vi "SMU calibration_Manual.vi"() -> ()   [LabVIEW 2020]
uses:
  <vilib>/Instr/_visa.llb/VISA Configure Serial Port (Instr).vi
  <vilib>/Analysis/NI_AALPro.lvlib
panel:
  out "output cal":dbl
  out "NewVal":bool
  out "tmp data":string
  out "Array":T1(array[cluster]) {"Output level" format="%.7f"; "Voltage" format="%.7f"; "Measurement" format="%.7f"}
  out "Array 3":bool[](array[boolean])
  out "Array 2":i32[](array[numeric])
  out "Unit":string
  in  "Output Value":dbl format="%.3f"
  in  "set Output":bool
  in  "Range":u16(ring) items=["1A", "100mA", "10mA", "1mA", "100uA", "10uA", "1uA"]
  in  "set range":bool
  in  "set mode":bool
  in  "Mode":bool
  out "test":bool
  out "extra buffer":string
  out "Write mode":bool
  in  "Enable":bool
  in  "Ring":u16(ring)=1 items=["Channel 1"=1, "Channel 2"=2, "Channel 3"=3, "Channel 4"=4]
  out "Range":string
  out "VI mode":string
  out "Enable":string
  out "Current":dbl
  out "Voltage":dbl
  out "Output level":dbl
  out "SMU Channel":string
  out "read buffer":string
  in  "VISA resource name":refnum<visa-resource-name>
  in  "stop":bool
  in  "set En":bool
  in  "String":string
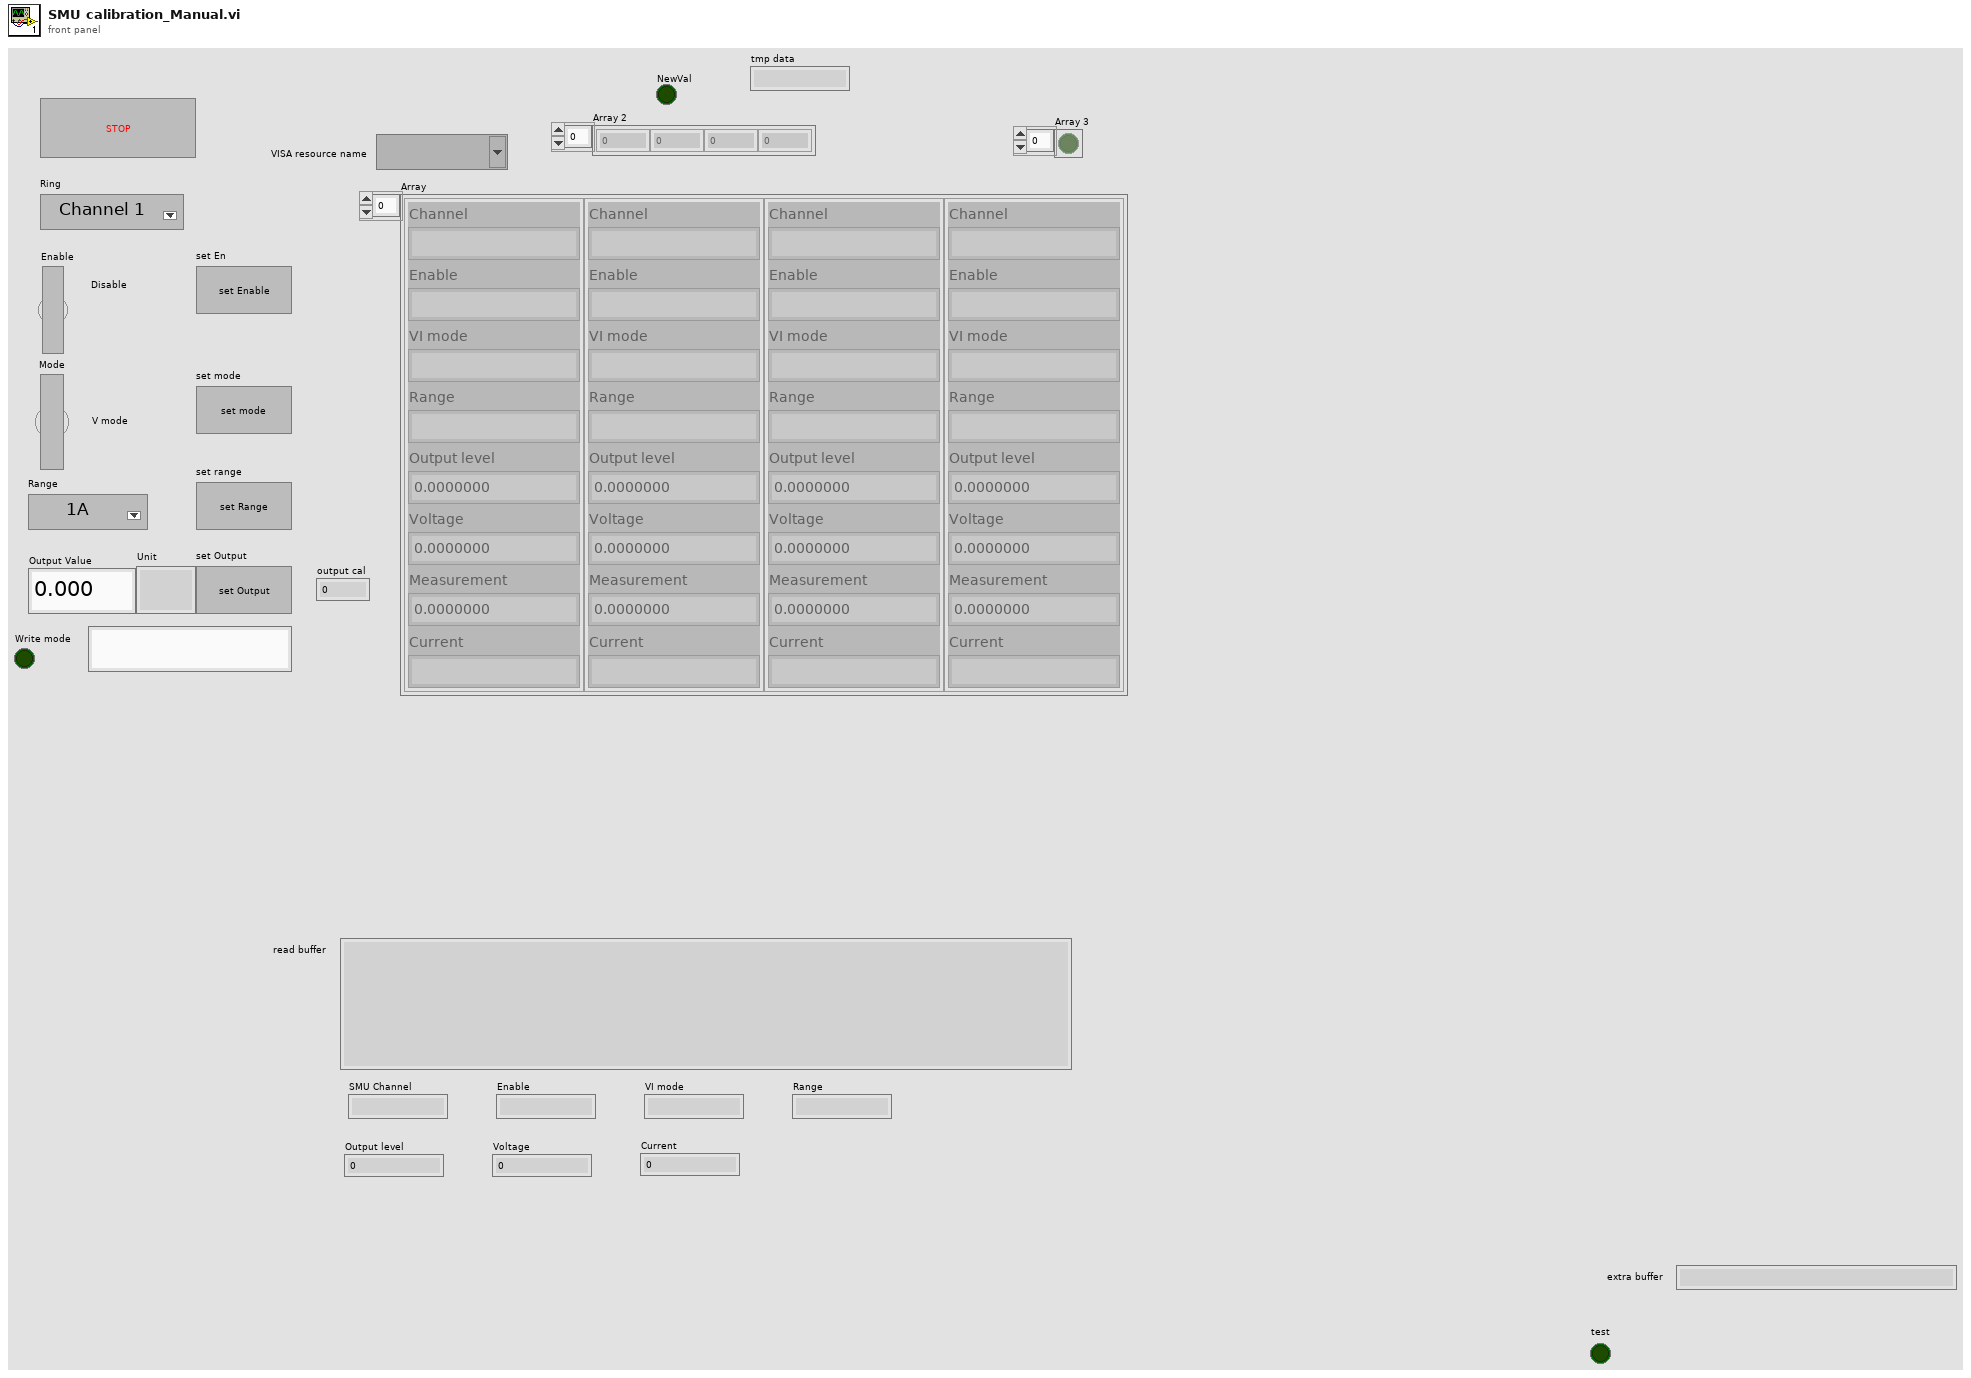
[diagram p1: front panel]
types:
  T1 = cluster{"Channel":string, "Enable":string, "VI mode":string, "Range":string, "Output level":dbl, "Voltage":dbl, "Measurement":dbl, "Current":string}[]
  T2 = cluster{"trimmed string":string, "Enable":string, "VI mode":string, "output string":string, dbl, dbl, dbl, string}
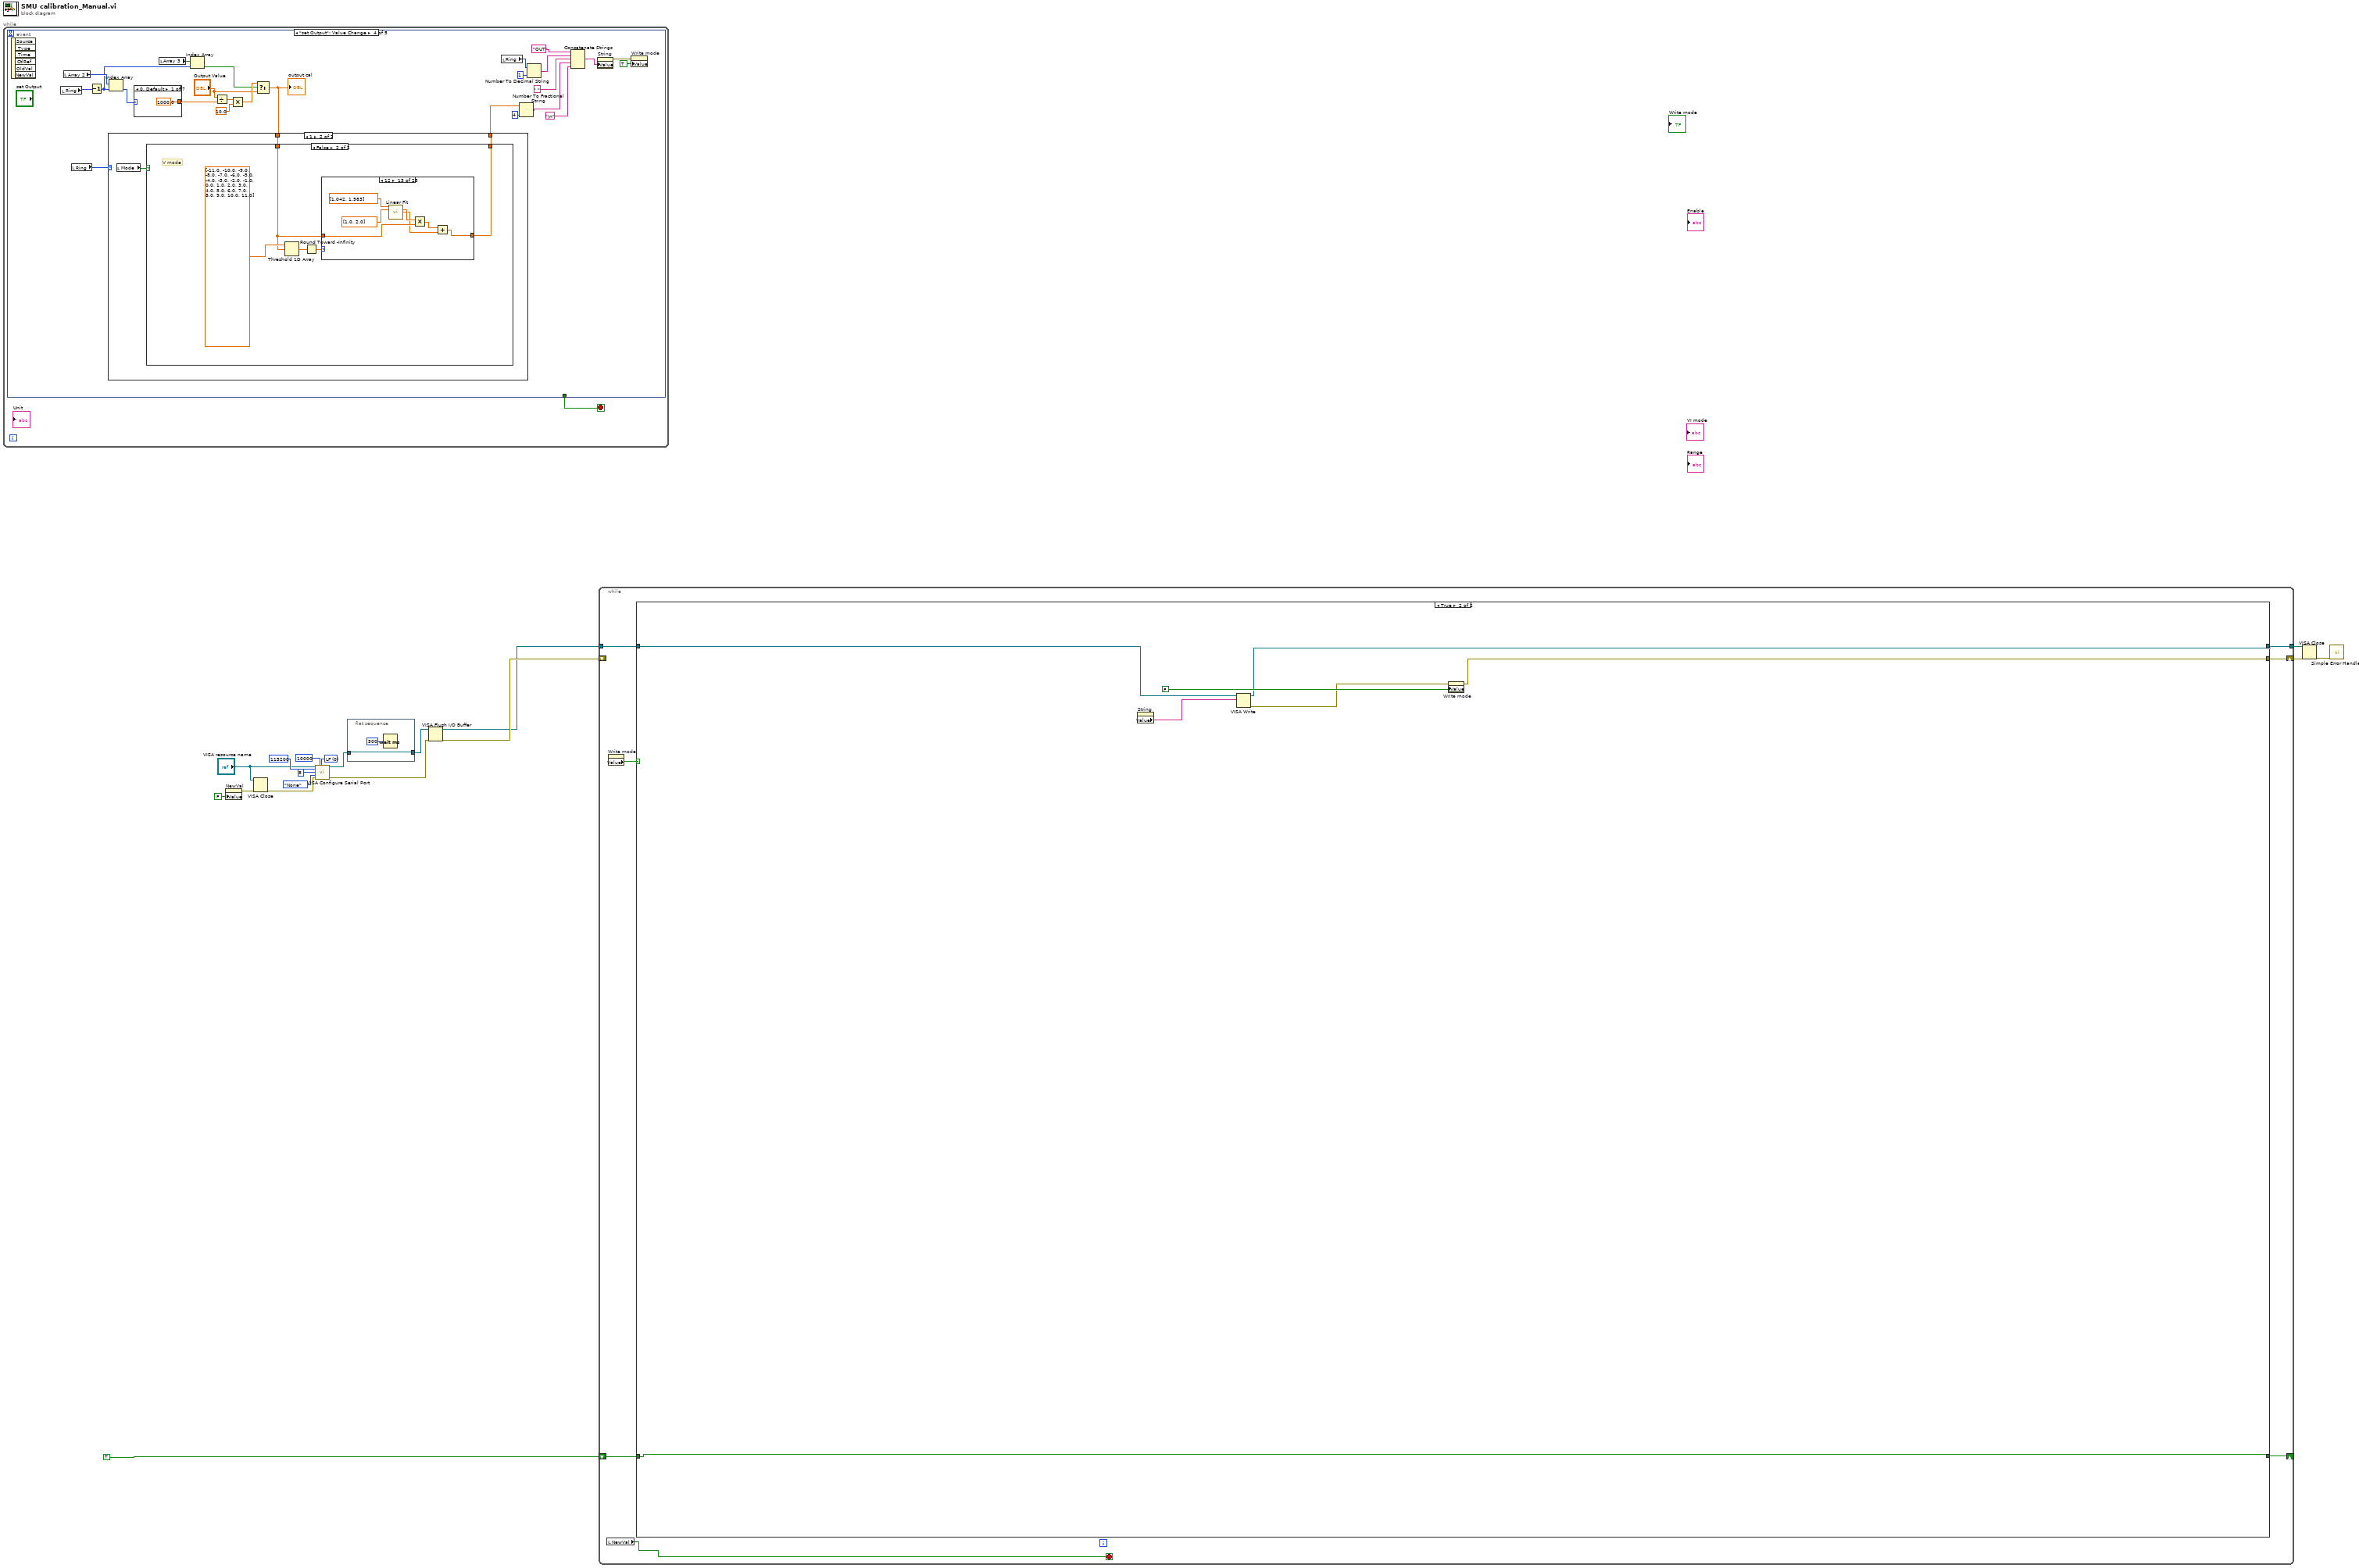
[diagram p0: block diagram]
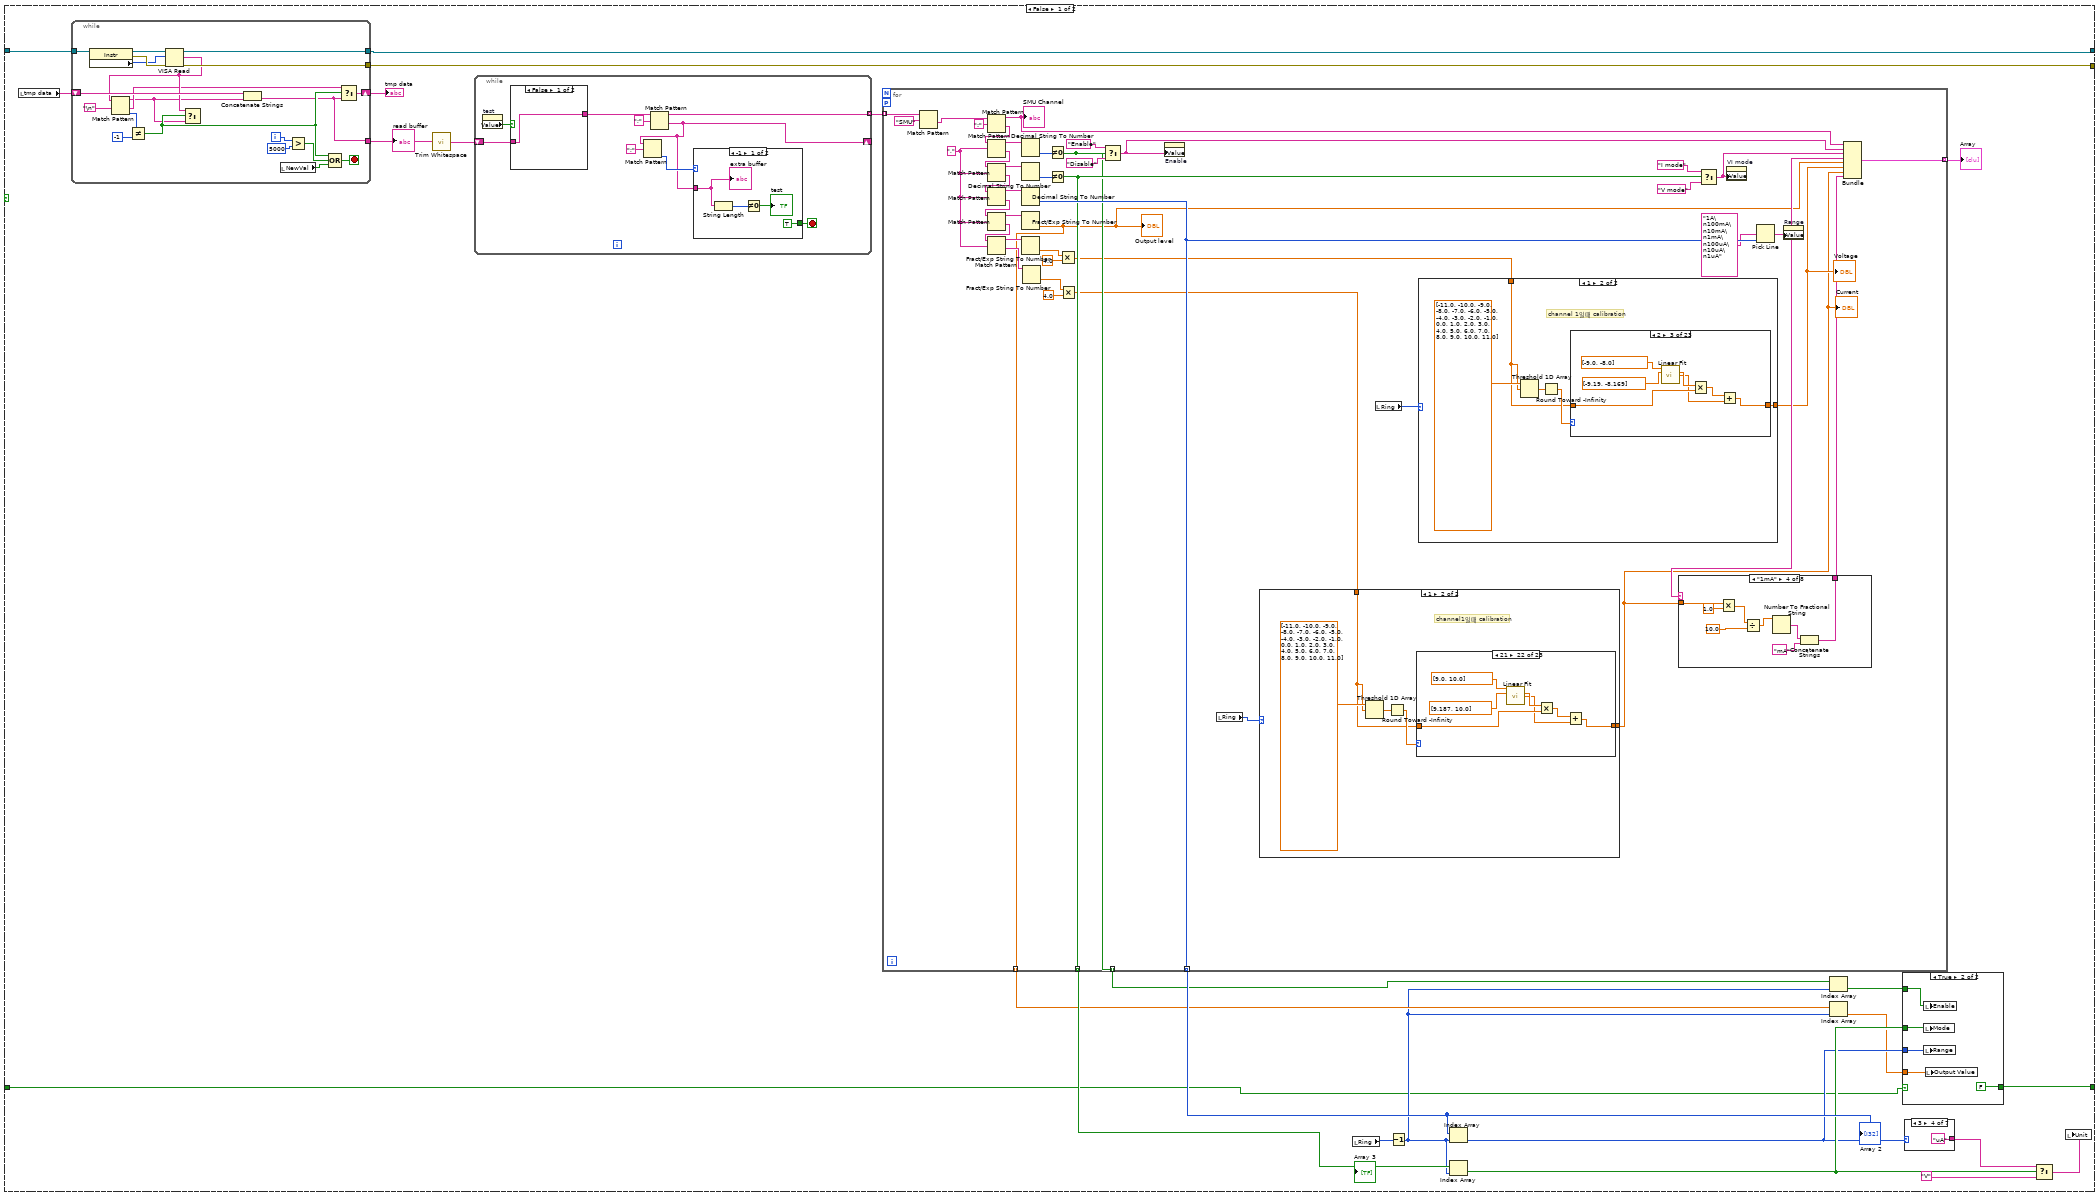
[diagram p2: hidden frame]
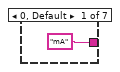
[diagram p4: hidden frame]
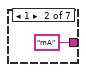
[diagram p5: hidden frame]
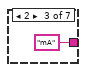
[diagram p6: hidden frame]
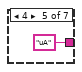
[diagram p7: hidden frame]
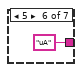
[diagram p8: hidden frame]
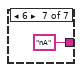
[diagram p9: hidden frame]
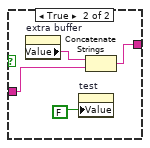
[diagram p10: hidden frame]
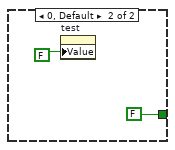
[diagram p11: hidden frame]
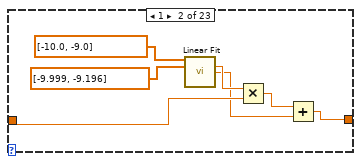
[diagram p14: hidden frame]
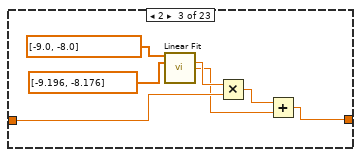
[diagram p15: hidden frame]
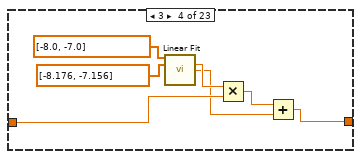
[diagram p16: hidden frame]
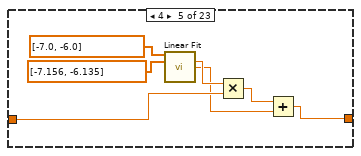
[diagram p17: hidden frame]
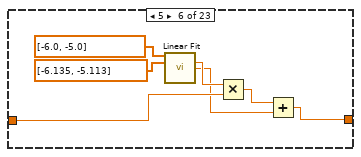
[diagram p18: hidden frame]
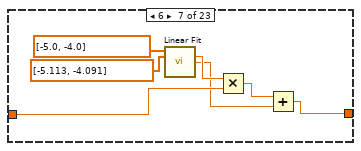
[diagram p19: hidden frame]
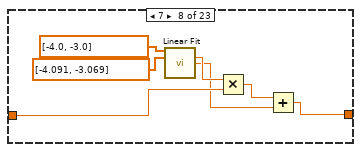
[diagram p20: hidden frame]
diagram:
  w16 = u16 0 items=["LF"]
  n1 = while {
    stop <- w19 stop-if-true
    n2 = event shown="[3] \"set Output\": Value Change" {
      selector: _ -> [_ _ _ _ _]
      dyn-events: _ -> [_ _ _ _ _]
      timeout: _ -> [_ _ _ _ _]
      tunnel: [_ _ _ _ w395] -> w19
      event "set En": Value Change {
        n3 = event-data() -> ()  [unwired: 1 in, 6 out]
        n4 = Boolean To (0,1)(Boolean="Enable") -> (0, 1=w31:i16)
        n5 = Number To Decimal String(number="Ring", width (-)=i16 1) -> (decimal integer string=w29:string)
        n6 = Number To Decimal String(number=w31, width (-)=i16 1) -> (decimal integer string=w32:string)
        n7 = Concatenate Strings("ENA", w29, " " ("string"), w32, "\n") -> (w20:string)
        n8 = property on="String" class="Str"("Value"=w20) -> (error out=w22:errorcluster)  [unwired: 2 in, 1 out]
        n9 = property on="Write mode" class="Bool (strict)"(error in=w22, "Value"=TRUE ("Write mode")) -> ()  [unwired: 1 in, 2 out]
      }
      event "set mode": Value Change {
        n10 = event-data() -> ()  [unwired: 1 in, 6 out]
        n11 = local read "Ring"() -> (w45:u16)
        n12 = Boolean To (0,1)(Boolean="Mode") -> (0, 1=w43:i16)
        n13 = Number To Decimal String(number=w45, width (-)=i16 1) -> (decimal integer string=w41:string)
        n14 = Number To Decimal String(number=w43, width (-)=i16 1) -> (decimal integer string=w44:string)
        n15 = Concatenate Strings("VIM", w41, " " ("string"), w44, "\n") -> (w39:string)
        n16 = property on="String" class="Str"("Value"=w39) -> (error out=w40:errorcluster)  [unwired: 2 in, 1 out]
        n17 = property on="Write mode" class="Bool (strict)"(error in=w40, "Value"=TRUE ("Write mode")) -> ()  [unwired: 1 in, 2 out]
      }
      event "set range": Value Change {
        n18 = event-data() -> ()  [unwired: 1 in, 6 out]
        n19 = local read "Ring"() -> (w56:u16)
        n20 = Number To Decimal String(number=w56, width (-)=i16 1) -> (decimal integer string=w54:string)
        n21 = Number To Decimal String(number="Range", width (-)=i16 1) -> (decimal integer string=w55:string)
        n22 = Concatenate Strings("RAN", w54, " " ("string"), w55, "\n") -> (w52:string)
        n23 = property on="String" class="Str"("Value"=w52) -> (error out=w53:errorcluster)  [unwired: 2 in, 1 out]
        n24 = property on="Write mode" class="Bool (strict)"(error in=w53, "Value"=TRUE ("Write mode")) -> ()  [unwired: 1 in, 2 out]
      }
      event "set Output": Value Change {
        n25 = event-data() -> ()  [unwired: 1 in, 6 out]
        n26 = local read "Ring"() -> (w68:u16)
        n27 = local read "Array 2"() -> (w67:i32[])
        n28 = local read "Ring"() -> (w58:u16)
        n29 = Decrement(x=w68) -> (x-1=w61:u16)
        n30 = Index Array(array=w67, index=w61) -> (element=w66:i32)
        n31 = case shown="0, Default" w66 {
          tunnel: [1000.0 100.0 10.0 1000.0 100.0 10.0 1.0] -> w69
          frame 0, Default {
          }
          frame 1 {
          }
          frame 2 {
          }
          frame 3 {
          }
          frame 4 {
          }
          frame 5 {
          }
          frame 6 {
          }
        }
        n32 = local read "Array 3"() -> (w63:bool[])
        n33 = Index Array(array=w63, index=w61) -> (element=w62:bool)
        n34 = Divide(x="Output Value", y=w69) -> (x/y=w70:dbl)
        n35 = Multiply(x=w70, y=10.0) -> (x*y=w65:dbl)
        n36 = Select(t=w65, s=w62, f="Output Value") -> (s? t:f=w60:dbl)
        "output cal" <- w60
        n37 = case shown="1" w58 {
          tunnel: w60 -> [w83 w86]
          tunnel: [w83 w85] -> w59
          frame 0, Default {
          }
          frame 1 {
            n38 = local read "Mode"() -> (w84:bool)
            n39 = case shown="False" w84 {
              tunnel: w86 -> [w88 w235]
              tunnel: [w87 w234] -> w85
              frame True {
                # "I mode"
                n40 = local read "Range"() -> (w89:u16)
                n41 = case shown="1" w89 {
                  tunnel: w88 -> [w90 w95 w119 w148 w177 w206]
                  tunnel: [w90 w94 w118 w147 w176 w205] -> w87
                  frame 0, Default {
                  }
                  frame 1 {
                    # "100mA일 경우"
                    n42 = Threshold 1D Array(2:w95, 3:dbl[] [-4.0, -3.5, -3.0, -2.0, -1.0, 0.0, 1.0, 2.0, 3.0, 4.0, 5.0, 6.0, 6.0]) -> (0:w92:dbl)  [unwired: 1 in]
                    n43 = Round Toward -Infinity(1:w92) -> (0:w91:dbl)
                    n44 = case shown="7" w91 {
                      tunnel: w95 -> [w96 w98 w100 w102 w104 w106 w108 w110 w112 w114 w116 w117]
                      tunnel: [w96 w97 w99 w101 w103 w105 w107 w109 w111 w113 w115 w117] -> w94
                      frame 0, Default {
                      }
                      frame 1 {
                        n45 = expression code="1.07 *x - 0.014"(w98) -> (w97:dbl)
                      }
                      frame 2 {
                        n46 = expression code="1.071* x - 0.011"(w100) -> (w99:dbl)
                      }
                      frame 3 {
                        n47 = expression code="1.071 *x - 0.011"(w102) -> (w101:dbl)
                      }
                      frame 4 {
                        n48 = expression code="1.075 * x - 0.007"(w104) -> (w103:dbl)
                      }
                      frame 5 {
                        n49 = expression code="1.069 *x - 0.007"(w106) -> (w105:dbl)
                      }
                      frame 6 {
                        n50 = expression code="1.071* x - 0.009"(w108) -> (w107:dbl)
                      }
                      frame 7 {
                        n51 = expression code="1.07* x - 0.007"(w110) -> (w109:dbl)
                      }
                      frame 8 {
                        n52 = expression code="1.069 *x - 0.004"(w112) -> (w111:dbl)
                      }
                      frame 9 {
                        n53 = expression code="1.07 *x - 0.008"(w114) -> (w113:dbl)
                      }
                      frame 10 {
                        n54 = expression code="1.07 *x - 0.008"(w116) -> (w115:dbl)
                      }
                      frame 11 {
                      }
                    }
                  }
                  frame 2 {
                    # "10mA일 경우"
                    n55 = Threshold 1D Array(2:w119, 3:dbl[] [-6.0, -5.0, -4.0, -3.0, -2.0, -1.0, 0.0, 1.0, 2.0, 3.0, 4.0, 5.0, 6.0]) -> (0:w122:dbl)  [unwired: 1 in]
                    n56 = Round Toward -Infinity(1:w122) -> (0:w121:dbl)
                    n57 = case shown="0, Default" w121 {
                      tunnel: w119 -> [w123 w125 w127 w129 w131 w133 w135 w137 w139 w141 w143 w145 w146]
                      tunnel: [w123 w124 w126 w128 w130 w132 w134 w136 w138 w140 w142 w144 w146] -> w118
                      frame 0, Default {
                      }
                      frame 1 {
                        n58 = expression code="1.043 * x - 0.01"(w125) -> (w124:dbl)
                      }
                      frame 2 {
                        n59 = expression code="1.043 * x - 0.01"(w127) -> (w126:dbl)
                      }
                      frame 3 {
                        n60 = expression code="1.042 * x - 0.013"(w129) -> (w128:dbl)
                      }
                      frame 4 {
                        n61 = expression code="1.043 * x - 0.011"(w131) -> (w130:dbl)
                      }
                      frame 5 {
                        n62 = expression code="1.044 * x - 0.01"(w133) -> (w132:dbl)
                      }
                      frame 6 {
                        n63 = expression code="1.045 * x - 0.01"(w135) -> (w134:dbl)
                      }
                      frame 7 {
                        n64 = expression code="1.042 * x - 0.007"(w137) -> (w136:dbl)
                      }
                      frame 8 {
                        n65 = expression code="1.043 * x - 0.009"(w139) -> (w138:dbl)
                      }
                      frame 9 {
                        n66 = expression code="1.042 * x - 0.006"(w141) -> (w140:dbl)
                      }
                      frame 10 {
                        n67 = expression code="1.041 * x - 0.002"(w143) -> (w142:dbl)
                      }
                      frame 11 {
                        n68 = expression code="1.043 * x - 0.012"(w145) -> (w144:dbl)
                      }
                      frame 12 {
                      }
                    }
                  }
                  frame 3 {
                    # "1mA 경우"
                    n69 = Threshold 1D Array(2:w148, 3:dbl[] [-6.0, -5.0, -4.0, -3.0, -2.0, -1.0, 0.0, 1.0, 2.0, 3.0, 4.0, 5.0, 6.0]) -> (0:w151:dbl)  [unwired: 1 in]
                    n70 = Round Toward -Infinity(1:w151) -> (0:w150:dbl)
                    n71 = case shown="12" w150 {
                      tunnel: w148 -> [w152 w154 w156 w158 w160 w162 w164 w166 w168 w170 w172 w174 w175]
                      tunnel: [w152 w153 w155 w157 w159 w161 w163 w165 w167 w169 w171 w173 w175] -> w147
                      frame 0, Default {
                      }
                      frame 1 {
                        n72 = expression code="1.043 *x - 0.009"(w154) -> (w153:dbl)
                      }
                      frame 2 {
                        n73 = expression code="1.042 *x - 0.013"(w156) -> (w155:dbl)
                      }
                      frame 3 {
                        n74 = expression code="1.042 *x - 0.013"(w158) -> (w157:dbl)
                      }
                      frame 4 {
                        n75 = expression code="1.043* x - 0.011"(w160) -> (w159:dbl)
                      }
                      frame 5 {
                        n76 = expression code="1.042* x - 0.012"(w162) -> (w161:dbl)
                      }
                      frame 6 {
                        n77 = expression code="1.046 *x - 0.012"(w164) -> (w163:dbl)
                      }
                      frame 7 {
                        n78 = expression code="1.042 *x - 0.008"(w166) -> (w165:dbl)
                      }
                      frame 8 {
                        n79 = expression code="1.042 *x - 0.008"(w168) -> (w167:dbl)
                      }
                      frame 9 {
                        n80 = expression code="1.043 *x - 0.011"(w170) -> (w169:dbl)
                      }
                      frame 10 {
                        n81 = expression code="1.041 *x - 0.003"(w172) -> (w171:dbl)
                      }
                      frame 11 {
                        n82 = expression code="1.042 *x - 0.008"(w174) -> (w173:dbl)
                      }
                      frame 12 {
                      }
                    }
                  }
                  frame 4 {
                    # "100uA 경우"
                    n83 = Threshold 1D Array(2:w177, 3:dbl[] [-6.0, -5.0, -4.0, -3.0, -2.0, -1.0, 0.0, 1.0, 2.0, 3.0, 4.0, 5.0, 6.0]) -> (0:w180:dbl)  [unwired: 1 in]
                    n84 = Round Toward -Infinity(1:w180) -> (0:w179:dbl)
                    n85 = case shown="12" w179 {
                      tunnel: w177 -> [w181 w183 w185 w187 w189 w191 w193 w195 w197 w199 w201 w203 w204]
                      tunnel: [w181 w182 w184 w186 w188 w190 w192 w194 w196 w198 w200 w202 w204] -> w176
                      frame 0, Default {
                      }
                      frame 1 {
                        n86 = expression code="1.046 *x - 0.001"(w183) -> (w182:dbl)
                      }
                      frame 2 {
                        n87 = expression code="1.042* x - 0.017"(w185) -> (w184:dbl)
                      }
                      frame 3 {
                        n88 = expression code="1.044 *x - 0.011"(w187) -> (w186:dbl)
                      }
                      frame 4 {
                        n89 = expression code="1.042 *x - 0.015"(w189) -> (w188:dbl)
                      }
                      frame 5 {
                        n90 = expression code="1.043* x - 0.014"(w191) -> (w190:dbl)
                      }
                      frame 6 {
                        n91 = expression code="1.043* x - 0.014"(w193) -> (w192:dbl)
                      }
                      frame 7 {
                        n92 = expression code="1.042 *x - 0.013"(w195) -> (w194:dbl)
                      }
                      frame 8 {
                        n93 = expression code="1.041* x - 0.011"(w197) -> (w196:dbl)
                      }
                      frame 9 {
                        n94 = expression code="1.041* x - 0.011"(w199) -> (w198:dbl)
                      }
                      frame 10 {
                        n95 = expression code="1.041* x - 0.011"(w201) -> (w200:dbl)
                      }
                      frame 11 {
                        n96 = expression code="1.042 *x - 0.008"(w203) -> (w202:dbl)
                      }
                      frame 12 {
                      }
                    }
                  }
                  frame 5 {
                    # "10uA 경우"
                    n97 = Threshold 1D Array(2:w206, 3:dbl[] [-6.0, -5.0, -4.0, -3.0, -2.0, -1.0, 0.0, 1.0, 2.0, 3.0, 4.0, 5.0, 6.0]) -> (0:w209:dbl)  [unwired: 1 in]
                    n98 = Round Toward -Infinity(1:w209) -> (0:w208:dbl)
                    n99 = case shown="12" w208 {
                      tunnel: w206 -> [w210 w212 w214 w216 w218 w220 w222 w224 w226 w228 w230 w232 w233]
                      tunnel: [w210 w211 w213 w215 w217 w219 w221 w223 w225 w227 w229 w231 w233] -> w205
                      frame 0, Default {
                      }
                      frame 1 {
                        n100 = expression code="1.045* x - 0.05"(w212) -> (w211:dbl)
                      }
                      frame 2 {
                        n101 = expression code="1.045 *x - 0.05"(w214) -> (w213:dbl)
                      }
                      frame 3 {
                        n102 = expression code="1.055 *x - 0.02"(w216) -> (w215:dbl)
                      }
                      frame 4 {
                        n103 = expression code="1.041 *x - 0.048"(w218) -> (w217:dbl)
                      }
                      frame 5 {
                        n104 = expression code="1.039 *x - 0.05"(w220) -> (w219:dbl)
                      }
                      frame 6 {
                        n105 = expression code="1.048 *x - 0.05"(w222) -> (w221:dbl)
                      }
                      frame 7 {
                        n106 = expression code="1.039* x - 0.041"(w224) -> (w223:dbl)
                      }
                      frame 8 {
                        n107 = expression code="1.045* x - 0.053"(w226) -> (w225:dbl)
                      }
                      frame 9 {
                        n108 = expression code="1.039 *x - 0.035"(w228) -> (w227:dbl)
                      }
                      frame 10 {
                        n109 = expression code="1.034 *x - 0.015"(w230) -> (w229:dbl)
                      }
                      frame 11 {
                        n110 = expression code="1.054* x - 0.115"(w232) -> (w231:dbl)
                      }
                      frame 12 {
                      }
                    }
                  }
                }
              }
              frame False {
                # "V mode"
                n111 = Threshold 1D Array(2:w235, 3:dbl[] [-11.0, -10.0, -9.0, -8.0, -7.0, -6.0, -5.0, -4.0, -3.0, -2.0, -1.0, 0.0, 1.0, 2.0, 3.0, 4.0, 5.0, 6.0, 7.0, 8.0, 9.0, 10.0, 11.0]) -> (0:w238:dbl)  [unwired: 1 in]
                n112 = Round Toward -Infinity(1:w238) -> (0:w236:dbl)
                n113 = case shown="12" w236 {
                  tunnel: w235 -> [w239 w245 w252 w259 w266 w273 w280 w287 w294 w301 w306 w313 w320 w327 w334 w341 w348 w355 w362 w369 w376 w383 w387]
                  tunnel: [w239 w242 w249 w256 w263 w270 w277 w284 w291 w298 w303 w310 w317 w324 w331 w338 w345 w352 w359 w366 w373 w380 w387] -> w234
                  frame 0, Default {
                  }
                  frame 1 {
                    n114 = call <vilib>:"Linear Fit.vi"("Y"=dbl[] [-9.308, -8.367], "X"=dbl[] [-10.0, -9.0]) -> ("slope"=w246:dbl, "intercept"=w244:dbl)  [unwired: 9 in, 3 out]
                    n115 = Multiply(x=w246, y=w245) -> (x*y=w243:dbl)
                    n116 = Add(x=w243, y=w244) -> (x+y=w242:dbl)
                  }
                  frame 2 {
                    n117 = call <vilib>:"Linear Fit.vi"("Y"=dbl[] [-8.367, -7.427], "X"=dbl[] [-9.0, -8.0]) -> ("slope"=w253:dbl, "intercept"=w251:dbl)  [unwired: 9 in, 3 out]
                    n118 = Multiply(x=w253, y=w252) -> (x*y=w250:dbl)
                    n119 = Add(x=w250, y=w251) -> (x+y=w249:dbl)
                  }
                  frame 3 {
                    n120 = call <vilib>:"Linear Fit.vi"("Y"=dbl[] [-7.427, -6.486], "X"=dbl[] [-8.0, -7.0]) -> ("slope"=w260:dbl, "intercept"=w258:dbl)  [unwired: 9 in, 3 out]
                    n121 = Multiply(x=w260, y=w259) -> (x*y=w257:dbl)
                    n122 = Add(x=w257, y=w258) -> (x+y=w256:dbl)
                  }
                  frame 4 {
                    n123 = call <vilib>:"Linear Fit.vi"("Y"=dbl[] [-6.486, -5.545], "X"=dbl[] [-7.0, -6.0]) -> ("slope"=w267:dbl, "intercept"=w265:dbl)  [unwired: 9 in, 3 out]
                    n124 = Multiply(x=w267, y=w266) -> (x*y=w264:dbl)
                    n125 = Add(x=w264, y=w265) -> (x+y=w263:dbl)
                  }
                  frame 5 {
                    n126 = call <vilib>:"Linear Fit.vi"("Y"=dbl[] [-5.545, -4.604], "X"=dbl[] [-6.0, -5.0]) -> ("slope"=w274:dbl, "intercept"=w272:dbl)  [unwired: 9 in, 3 out]
                    n127 = Multiply(x=w274, y=w273) -> (x*y=w271:dbl)
                    n128 = Add(x=w271, y=w272) -> (x+y=w270:dbl)
                  }
                  frame 6 {
                    n129 = call <vilib>:"Linear Fit.vi"("Y"=dbl[] [-4.604, -3.664], "X"=dbl[] [-5.0, -4.0]) -> ("slope"=w281:dbl, "intercept"=w279:dbl)  [unwired: 9 in, 3 out]
                    n130 = Multiply(x=w281, y=w280) -> (x*y=w278:dbl)
                    n131 = Add(x=w278, y=w279) -> (x+y=w277:dbl)
                  }
                  frame 7 {
                    n132 = call <vilib>:"Linear Fit.vi"("Y"=dbl[] [-3.664, -2.723], "X"=dbl[] [-4.0, -3.0]) -> ("slope"=w288:dbl, "intercept"=w286:dbl)  [unwired: 9 in, 3 out]
                    n133 = Multiply(x=w288, y=w287) -> (x*y=w285:dbl)
                    n134 = Add(x=w285, y=w286) -> (x+y=w284:dbl)
                  }
                  frame 8 {
                    n135 = call <vilib>:"Linear Fit.vi"("Y"=dbl[] [-2.723, -1.782], "X"=dbl[] [-3.0, -2.0]) -> ("slope"=w295:dbl, "intercept"=w293:dbl)  [unwired: 9 in, 3 out]
                    n136 = Multiply(x=w295, y=w294) -> (x*y=w292:dbl)
                    n137 = Add(x=w292, y=w293) -> (x+y=w291:dbl)
                  }
                  frame 9 {
                    n138 = call <vilib>:"Linear Fit.vi"("Y"=dbl[] [-1.782, -0.841], "X"=dbl[] [-2.0, -1.0]) -> ("slope"=w302:dbl, "intercept"=w300:dbl)  [unwired: 9 in, 3 out]
                    n139 = Multiply(x=w302, y=w301) -> (x*y=w299:dbl)
                    n140 = Add(x=w299, y=w300) -> (x+y=w298:dbl)
                  }
                  frame 10 {
                    n141 = call <vilib>:"Linear Fit.vi"("Y"=dbl[] [-0.841, 0.1], "X"=dbl[] [-1.0, 0.0]) -> ("slope"=w307:dbl, "intercept"=w305:dbl)  [unwired: 9 in, 3 out]
                    n142 = Multiply(x=w307, y=w306) -> (x*y=w304:dbl)
                    n143 = Add(x=w304, y=w305) -> (x+y=w303:dbl)
                  }
                  frame 11 {
                    n144 = call <vilib>:"Linear Fit.vi"("Y"=dbl[] [0.1, 1.042], "X"=dbl[] [0.0, 1.0]) -> ("slope"=w314:dbl, "intercept"=w312:dbl)  [unwired: 9 in, 3 out]
                    n145 = Multiply(x=w314, y=w313) -> (x*y=w311:dbl)
                    n146 = Add(x=w311, y=w312) -> (x+y=w310:dbl)
                  }
                  frame 12 {
                    n147 = call <vilib>:"Linear Fit.vi"("Y"=dbl[] [1.042, 1.983], "X"=dbl[] [1.0, 2.0]) -> ("slope"=w321:dbl, "intercept"=w319:dbl)  [unwired: 9 in, 3 out]
                    n148 = Multiply(x=w321, y=w320) -> (x*y=w318:dbl)
                    n149 = Add(x=w318, y=w319) -> (x+y=w317:dbl)
                  }
                  frame 13 {
                    n150 = call <vilib>:"Linear Fit.vi"("Y"=dbl[] [1.983, 2.924], "X"=dbl[] [2.0, 3.0]) -> ("slope"=w328:dbl, "intercept"=w326:dbl)  [unwired: 9 in, 3 out]
                    n151 = Multiply(x=w328, y=w327) -> (x*y=w325:dbl)
                    n152 = Add(x=w325, y=w326) -> (x+y=w324:dbl)
                  }
                  frame 14 {
                    n153 = call <vilib>:"Linear Fit.vi"("Y"=dbl[] [2.924, 3.864], "X"=dbl[] [3.0, 4.0]) -> ("slope"=w335:dbl, "intercept"=w333:dbl)  [unwired: 9 in, 3 out]
                    n154 = Multiply(x=w335, y=w334) -> (x*y=w332:dbl)
                    n155 = Add(x=w332, y=w333) -> (x+y=w331:dbl)
                  }
                  frame 15 {
                    n156 = call <vilib>:"Linear Fit.vi"("Y"=dbl[] [3.864, 4.804], "X"=dbl[] [4.0, 5.0]) -> ("slope"=w342:dbl, "intercept"=w340:dbl)  [unwired: 9 in, 3 out]
                    n157 = Multiply(x=w342, y=w341) -> (x*y=w339:dbl)
                    n158 = Add(x=w339, y=w340) -> (x+y=w338:dbl)
                  }
                  frame 16 {
                    n159 = call <vilib>:"Linear Fit.vi"("Y"=dbl[] [4.804, 5.745], "X"=dbl[] [5.0, 6.0]) -> ("slope"=w349:dbl, "intercept"=w347:dbl)  [unwired: 9 in, 3 out]
                    n160 = Multiply(x=w349, y=w348) -> (x*y=w346:dbl)
                    n161 = Add(x=w346, y=w347) -> (x+y=w345:dbl)
                  }
                  frame 17 {
                    n162 = call <vilib>:"Linear Fit.vi"("Y"=dbl[] [5.745, 6.686], "X"=dbl[] [6.0, 7.0]) -> ("slope"=w356:dbl, "intercept"=w354:dbl)  [unwired: 9 in, 3 out]
                    n163 = Multiply(x=w356, y=w355) -> (x*y=w353:dbl)
                    n164 = Add(x=w353, y=w354) -> (x+y=w352:dbl)
                  }
                  frame 18 {
                    n165 = call <vilib>:"Linear Fit.vi"("Y"=dbl[] [6.686, 7.627], "X"=dbl[] [7.0, 8.0]) -> ("slope"=w363:dbl, "intercept"=w361:dbl)  [unwired: 9 in, 3 out]
                    n166 = Multiply(x=w363, y=w362) -> (x*y=w360:dbl)
                    n167 = Add(x=w360, y=w361) -> (x+y=w359:dbl)
                  }
                  frame 19 {
                    n168 = call <vilib>:"Linear Fit.vi"("Y"=dbl[] [7.627, 8.567], "X"=dbl[] [8.0, 9.0]) -> ("slope"=w370:dbl, "intercept"=w368:dbl)  [unwired: 9 in, 3 out]
                    n169 = Multiply(x=w370, y=w369) -> (x*y=w367:dbl)
                    n170 = Add(x=w367, y=w368) -> (x+y=w366:dbl)
                  }
                  frame 20 {
                    n171 = call <vilib>:"Linear Fit.vi"("Y"=dbl[] [8.567, 9.507], "X"=dbl[] [9.0, 10.0]) -> ("slope"=w377:dbl, "intercept"=w375:dbl)  [unwired: 9 in, 3 out]
                    n172 = Multiply(x=w377, y=w376) -> (x*y=w374:dbl)
                    n173 = Add(x=w374, y=w375) -> (x+y=w373:dbl)
                  }
                  frame 21 {
                    n174 = call <vilib>:"Linear Fit.vi"("Y"=dbl[] [8.567, 9.507], "X"=dbl[] [9.0, 10.0]) -> ("slope"=w384:dbl, "intercept"=w382:dbl)  [unwired: 9 in, 3 out]
                    n175 = Multiply(x=w384, y=w383) -> (x*y=w381:dbl)
                    n176 = Add(x=w381, y=w382) -> (x+y=w380:dbl)
                  }
                  frame 22 {
                  }
                }
              }
            }
          }
        }
        n177 = local read "Ring"() -> (w81:u16)
        n178 = Number To Fractional String(number=w59, precision (6)=i16 4) -> (F-format string=w82:string)  [unwired: 2 in]
        n179 = Number To Decimal String(number=w81, width (-)=i16 1) -> (decimal integer string=w80:string)
        n180 = Concatenate Strings("OUT", w80, " " ("string"), w82, "\n") -> (w78:string)
        n181 = property on="String" class="Str"("Value"=w78) -> (error out=w79:errorcluster)  [unwired: 2 in, 1 out]
        n182 = property on="Write mode" class="Bool (strict)"(error in=w79, "Value"=TRUE ("Write mode")) -> ()  [unwired: 1 in, 2 out]
      }
      event "stop": Value Change {
        n183 = event-data() -> ("NewVal"=w395:bool)  [unwired: 1 in, 5 out]
        "NewVal" <- w395
      }
    }
  }
  n184 = property on="NewVal" class="Bool (strict)"("Value"=FALSE ("NewVal")) -> (error out=w2:errorcluster)  [unwired: 2 in, 1 out]
  n185 = VISA Close(VISA resource name="VISA resource name", error in (no error)=w2) -> (error out=w4:errorcluster)
  n186 = call-poly "VISA Configure Serial Port"("VISA resource name"="VISA resource name", "timeout (10sec)"=u32 10000, "termination char\n(0xA = '\\n' = LF)"=w16, "baud rate (9600)"=u32 115200, "data bits (8)"=u16 8, "parity (0:none)"=enum16{"None", "Odd", "Even", "Mark", "Space"}."None", "error in (no error)"=w4) -> ("VISA resource name out"=w10:refnum<visa-resource-name>, "error out"=w8:errorcluster)  [unwired: 7 in]
  n187 = flat-sequence {
    tunnel: [w396] -> w9
    tunnel: w10 -> [w396]
    frame #0 {
      n188 = Wait (ms)(milliseconds to wait=u32 500 ("대기 시간(ms)")) -> ()  [unwired: 1 out]
    }
  }
  n189 = VISA Flush I/O Buffer(VISA resource name=w9, error in (no error)=w8) -> (VISA resource name out=w6:refnum<visa-resource-name>, error out=w7:errorcluster)  [unwired: 1 in]
  n190 = while {
    tunnel: [w403] -> w18
    shift-right: [w404] -> w12
    shift-left: w7 -> [_]
    tunnel: w6 -> [w402]
    shift-right: [w399] -> _
    shift-left: TRUE -> [w400]
    stop <- w398 stop-if-true
    n191 = local read "NewVal"() -> (w398:bool)
    n192 = property on="Write mode" class="Bool (strict)"() -> ("Value"=w401:bool)  [unwired: 2 in, 2 out]
    n193 = case shown="True" w401 {
      tunnel: [w420 w894] -> w404
      tunnel: [w419 w895] -> w403
      tunnel: w402 -> [w421 w898]
      tunnel: w400 -> [w409 w893]
      tunnel: [w408 w893] -> w399
      frame False {
        n194 = local read "tmp data"() -> (w418:string)
        n195 = while {
          tunnel: w421 -> [w447]
          tunnel: [w455] -> w420
          tunnel: [w454] -> w419
          shift-right: [w453] -> w417
          shift-left: w418 -> [w452]
          tunnel: [w437] -> w406
          i -> [w450]
          stop <- w451 stop-if-true
          n196 = property class="Instr"(reference=w447) -> (reference out=w446:refnum<visa-resource-name>, error out=w445:errorcluster, "Serial Settings:Number of Bytes at Serial Port"=w444:u32)  [unwired: 1 in]
          n197 = VISA Read(VISA resource name=w446, byte count=w444, error in (no error)=w445) -> (VISA resource name out=w454:refnum<visa-resource-name>, read buffer=w439:string, error out=w455:errorcluster)  [unwired: 1 out]
          n198 = Match Pattern(string=w439, regular expression="\n") -> (before substring=w435:string, after substring=w438:string, offset past match=w442:i32)  [unwired: 1 in, 1 out]
          n199 = Not Equal?(x=w442, y=-1) -> (x != y?=w440:bool)
          n200 = Select(t=w439, s=w440, f=w435) -> ()  [unwired: 1 out]
          n201 = Concatenate Strings(w452, w435) -> (w437:string)
          n202 = local read "NewVal"() -> (w436:bool)
          n203 = Greater?(x=w450, y=5000) -> (0:w448:bool)
          n204 = Compound Arithmetic op=OR(w440, w448, w436) -> (w451:bool)
          n205 = Select(t=w438, s=w440, f=w437) -> (s? t:f=w453:string)
        }
        "read buffer" <- w406
        "tmp data" <- w417
        n206 = call <vilib>:"Trim Whitespace.vi"("string"=w406) -> ("trimmed string"=w407:string)  [unwired: 1 in]
        n207 = while {
          shift-right: [w463] -> _
          shift-left: w407 -> [w466]
          tunnel: [w470] -> w428 mode=indexing
          stop <- w464 stop-if-true
          n208 = property on="test" class="Bool (strict)"() -> ("Value"=w467:bool)  [unwired: 2 in, 2 out]
          n209 = case shown="False" w467 {
            tunnel: w466 -> [w472 w475]
            tunnel: [w472 w474] -> w465
            frame False {
            }
            frame True {
              n210 = property on="extra buffer" class="Str"() -> ("Value"=w476:string)  [unwired: 2 in, 2 out]
              n211 = property on="test" class="Bool (strict)"("Value"=FALSE) -> ()  [unwired: 2 in, 2 out]
              n212 = Concatenate Strings(w476, w475) -> (w474:string)
            }
          }
          n213 = Match Pattern(string=w465, regular expression=";" ("search string")) -> (before substring=w470:string, after substring=w463:string)  [unwired: 1 in, 2 out]
          n214 = Match Pattern(string=w463, regular expression=";" ("search string")) -> (offset past match=w468:i32)  [unwired: 1 in, 3 out]
          n215 = case shown="-1" w468 {
            tunnel: w463 -> [w479 _]
            tunnel: [TRUE FALSE] -> w464
            frame -1 {
              n216 = String Length(string=w479) -> (length=w478:i32)
              n217 = Not Equal To 0?(x=w478) -> (x != 0?=→"test":bool)
              "extra buffer" <- w479
            }
            frame 0, Default {
              n218 = property on="test" class="Bool (strict)"("Value"=FALSE) -> ()  [unwired: 2 in, 2 out]
            }
          }
        }
        n219 = for {
          tunnel: [w525] -> w405 mode=indexing
          tunnel: w428 -> [w500] mode=indexing
          workers-P: _ -> [_]
          tunnel: [w495] -> w426 mode=indexing
          tunnel: [w494] -> w425 mode=indexing
          tunnel: [w490] -> w416 mode=indexing
          tunnel: [w489] -> w412 mode=indexing
          w516 = "," ("search string")
          n220 = Match Pattern(string=w500, regular expression="SMU") -> (after substring=w522:string)  [unwired: 1 in, 3 out]
          n221 = Match Pattern(string=w522, regular expression=":" ("search string")) -> (before substring=w501:string, after substring=w521:string)  [unwired: 1 in, 2 out]
          "SMU Channel" <- w501
          n222 = Match Pattern(string=w521, regular expression=w516) -> (before substring=w515:string, after substring=w520:string)  [unwired: 1 in, 2 out]
          n223 = Match Pattern(string=w520, regular expression=w516) -> (before substring=w510:string, after substring=w518:string)  [unwired: 1 in, 2 out]
          n224 = Match Pattern(string=w518, regular expression=w516) -> (before substring=w511:string, after substring=w519:string)  [unwired: 1 in, 2 out]
          n225 = Match Pattern(string=w519, regular expression=w516) -> (before substring=w512:string, after substring=w517:string)  [unwired: 1 in, 2 out]
          n226 = Match Pattern(string=w517, regular expression=w516) -> (before substring=w513:string, after substring=w514:string)  [unwired: 1 in, 2 out]
          n227 = Decimal String To Number(string=w515) -> (number=w509:i32)  [unwired: 2 in, 1 out]
          n228 = Decimal String To Number(string=w510) -> (number=w508:i32)  [unwired: 2 in, 1 out]
          n229 = Decimal String To Number(string=w511) -> (number=w495:i32)  [unwired: 2 in, 1 out]
          n230 = Fract/Exp String To Number(string=w512) -> (number=w489:dbl)  [unwired: 3 in, 1 out]
          "Output level" <- w489
          n231 = Fract/Exp String To Number(string=w513) -> (number=w496:dbl)  [unwired: 3 in, 1 out]
          n232 = Fract/Exp String To Number(string=w514) -> (number=w497:dbl)  [unwired: 3 in, 1 out]
          n233 = Not Equal To 0?(x=w509) -> (x != 0?=w490:bool)
          n234 = Not Equal To 0?(x=w508) -> (x != 0?=w494:bool)
          n235 = Multiply(x=w496, y=4.0) -> (x*y=w487:dbl)
          n236 = Multiply(x=w497, y=4.0) -> (x*y=w485:dbl)
          n237 = Select(t="Enable" ("Enable"), s=w490, f="Disable" ("Enable")) -> (s? t:f=w503:string)
          n238 = property on="Enable" class="Str"("Value"=w503) -> ()  [unwired: 2 in, 2 out]
          n239 = local read "Ring"() -> (w483:u16)
          n240 = case shown="1" w483 {
            tunnel: [w526 w528] -> w486
            tunnel: w485 -> [w526 w527]
            frame 0, Default {
            }
            frame 1 {
              # "channel1일때 calibration"
              n241 = Threshold 1D Array(2:w527, 3:dbl[] [-11.0, -10.0, -9.0, -8.0, -7.0, -6.0, -5.0, -4.0, -3.0, -2.0, -1.0, 0.0, 1.0, 2.0, 3.0, 4.0, 5.0, 6.0, 7.0, 8.0, 9.0, 10.0, 11.0]) -> (0:w531:dbl)  [unwired: 1 in]
              n242 = Round Toward -Infinity(1:w531) -> (0:w529:dbl)
              n243 = case shown="21" w529 {
                tunnel: w527 -> [w532 w538 w545 w552 w559 w566 w573 w580 w587 w594 w599 w606 w613 w620 w627 w634 w641 w648 w655 w662 w669 w676 w680]
                tunnel: [w532 w535 w542 w549 w556 w563 w570 w577 w584 w591 w596 w603 w610 w617 w624 w631 w638 w645 w652 w659 w666 w673 w680] -> w528
                frame 0, Default {
                }
                frame 1 {
                  n244 = call <vilib>:"Linear Fit.vi"("Y"=dbl[] [-10.0, -9.0], "X"=dbl[] [-9.999, -9.196]) -> ("slope"=w539:dbl, "intercept"=w537:dbl)  [unwired: 9 in, 3 out]
                  n245 = Multiply(x=w539, y=w538) -> (x*y=w536:dbl)
                  n246 = Add(x=w536, y=w537) -> (x+y=w535:dbl)
                }
                frame 2 {
                  n247 = call <vilib>:"Linear Fit.vi"("Y"=dbl[] [-9.0, -8.0], "X"=dbl[] [-9.196, -8.176]) -> ("slope"=w546:dbl, "intercept"=w544:dbl)  [unwired: 9 in, 3 out]
                  n248 = Multiply(x=w546, y=w545) -> (x*y=w543:dbl)
                  n249 = Add(x=w543, y=w544) -> (x+y=w542:dbl)
                }
                frame 3 {
                  n250 = call <vilib>:"Linear Fit.vi"("Y"=dbl[] [-8.0, -7.0], "X"=dbl[] [-8.176, -7.156]) -> ("slope"=w553:dbl, "intercept"=w551:dbl)  [unwired: 9 in, 3 out]
                  n251 = Multiply(x=w553, y=w552) -> (x*y=w550:dbl)
                  n252 = Add(x=w550, y=w551) -> (x+y=w549:dbl)
                }
                frame 4 {
                  n253 = call <vilib>:"Linear Fit.vi"("Y"=dbl[] [-7.0, -6.0], "X"=dbl[] [-7.156, -6.135]) -> ("slope"=w560:dbl, "intercept"=w558:dbl)  [unwired: 9 in, 3 out]
                  n254 = Multiply(x=w560, y=w559) -> (x*y=w557:dbl)
                  n255 = Add(x=w557, y=w558) -> (x+y=w556:dbl)
                }
                frame 5 {
                  n256 = call <vilib>:"Linear Fit.vi"("Y"=dbl[] [-6.0, -5.0], "X"=dbl[] [-6.135, -5.113]) -> ("slope"=w567:dbl, "intercept"=w565:dbl)  [unwired: 9 in, 3 out]
                  n257 = Multiply(x=w567, y=w566) -> (x*y=w564:dbl)
                  n258 = Add(x=w564, y=w565) -> (x+y=w563:dbl)
                }
                frame 6 {
                  n259 = call <vilib>:"Linear Fit.vi"("Y"=dbl[] [-5.0, -4.0], "X"=dbl[] [-5.113, -4.091]) -> ("slope"=w574:dbl, "intercept"=w572:dbl)  [unwired: 9 in, 3 out]
                  n260 = Multiply(x=w574, y=w573) -> (x*y=w571:dbl)
                  n261 = Add(x=w571, y=w572) -> (x+y=w570:dbl)
                }
                frame 7 {
                  n262 = call <vilib>:"Linear Fit.vi"("Y"=dbl[] [-4.0, -3.0], "X"=dbl[] [-4.091, -3.069]) -> ("slope"=w581:dbl, "intercept"=w579:dbl)  [unwired: 9 in, 3 out]
                  n263 = Multiply(x=w581, y=w580) -> (x*y=w578:dbl)
                  n264 = Add(x=w578, y=w579) -> (x+y=w577:dbl)
                }
                frame 8 {
                  n265 = call <vilib>:"Linear Fit.vi"("Y"=dbl[] [-3.0, -2.0], "X"=dbl[] [-3.069, -2.047]) -> ("slope"=w588:dbl, "intercept"=w586:dbl)  [unwired: 9 in, 3 out]
                  n266 = Multiply(x=w588, y=w587) -> (x*y=w585:dbl)
                  n267 = Add(x=w585, y=w586) -> (x+y=w584:dbl)
                }
                frame 9 {
                  n268 = call <vilib>:"Linear Fit.vi"("Y"=dbl[] [-2.0, -1.0], "X"=dbl[] [-2.047, -1.025]) -> ("slope"=w595:dbl, "intercept"=w593:dbl)  [unwired: 9 in, 3 out]
                  n269 = Multiply(x=w595, y=w594) -> (x*y=w592:dbl)
                  n270 = Add(x=w592, y=w593) -> (x+y=w591:dbl)
                }
                frame 10 {
                  n271 = call <vilib>:"Linear Fit.vi"("Y"=dbl[] [-1.0, 0.0], "X"=dbl[] [-1.025, -0.003]) -> ("slope"=w600:dbl, "intercept"=w598:dbl)  [unwired: 9 in, 3 out]
                  n272 = Multiply(x=w600, y=w599) -> (x*y=w597:dbl)
                  n273 = Add(x=w597, y=w598) -> (x+y=w596:dbl)
                }
                frame 11 {
                  n274 = call <vilib>:"Linear Fit.vi"("Y"=dbl[] [0.0, 1.0], "X"=dbl[] [-0.003, 1.018]) -> ("slope"=w607:dbl, "intercept"=w605:dbl)  [unwired: 9 in, 3 out]
                  n275 = Multiply(x=w607, y=w606) -> (x*y=w604:dbl)
                  n276 = Add(x=w604, y=w605) -> (x+y=w603:dbl)
                }
                frame 12 {
                  n277 = call <vilib>:"Linear Fit.vi"("Y"=dbl[] [1.0, 2.0], "X"=dbl[] [1.018, 2.04]) -> ("slope"=w614:dbl, "intercept"=w612:dbl)  [unwired: 9 in, 3 out]
                  n278 = Multiply(x=w614, y=w613) -> (x*y=w611:dbl)
                  n279 = Add(x=w611, y=w612) -> (x+y=w610:dbl)
                }
                frame 13 {
                  n280 = call <vilib>:"Linear Fit.vi"("Y"=dbl[] [2.0, 3.0], "X"=dbl[] [2.04, 3.061]) -> ("slope"=w621:dbl, "intercept"=w619:dbl)  [unwired: 9 in, 3 out]
                  n281 = Multiply(x=w621, y=w620) -> (x*y=w618:dbl)
                  n282 = Add(x=w618, y=w619) -> (x+y=w617:dbl)
                }
                frame 14 {
                  n283 = call <vilib>:"Linear Fit.vi"("Y"=dbl[] [3.0, 4.0], "X"=dbl[] [3.061, 4.083]) -> ("slope"=w628:dbl, "intercept"=w626:dbl)  [unwired: 9 in, 3 out]
                  n284 = Multiply(x=w628, y=w627) -> (x*y=w625:dbl)
                  n285 = Add(x=w625, y=w626) -> (x+y=w624:dbl)
                }
                frame 15 {
                  n286 = call <vilib>:"Linear Fit.vi"("Y"=dbl[] [4.0, 5.0], "X"=dbl[] [4.083, 5.104]) -> ("slope"=w635:dbl, "intercept"=w633:dbl)  [unwired: 9 in, 3 out]
                  n287 = Multiply(x=w635, y=w634) -> (x*y=w632:dbl)
                  n288 = Add(x=w632, y=w633) -> (x+y=w631:dbl)
                }
                frame 16 {
                  n289 = call <vilib>:"Linear Fit.vi"("Y"=dbl[] [5.0, 6.0], "X"=dbl[] [5.104, 6.126]) -> ("slope"=w642:dbl, "intercept"=w640:dbl)  [unwired: 9 in, 3 out]
                  n290 = Multiply(x=w642, y=w641) -> (x*y=w639:dbl)
                  n291 = Add(x=w639, y=w640) -> (x+y=w638:dbl)
                }
                frame 17 {
                  n292 = call <vilib>:"Linear Fit.vi"("Y"=dbl[] [6.0, 7.0], "X"=dbl[] [6.126, 7.146]) -> ("slope"=w649:dbl, "intercept"=w647:dbl)  [unwired: 9 in, 3 out]
                  n293 = Multiply(x=w649, y=w648) -> (x*y=w646:dbl)
                  n294 = Add(x=w646, y=w647) -> (x+y=w645:dbl)
                }
                frame 18 {
                  n295 = call <vilib>:"Linear Fit.vi"("Y"=dbl[] [7.0, 8.0], "X"=dbl[] [7.146, 8.166]) -> ("slope"=w656:dbl, "intercept"=w654:dbl)  [unwired: 9 in, 3 out]
                  n296 = Multiply(x=w656, y=w655) -> (x*y=w653:dbl)
                  n297 = Add(x=w653, y=w654) -> (x+y=w652:dbl)
                }
                frame 19 {
                  n298 = call <vilib>:"Linear Fit.vi"("Y"=dbl[] [8.0, 9.0], "X"=dbl[] [8.166, 9.187]) -> ("slope"=w663:dbl, "intercept"=w661:dbl)  [unwired: 9 in, 3 out]
                  n299 = Multiply(x=w663, y=w662) -> (x*y=w660:dbl)
                  n300 = Add(x=w660, y=w661) -> (x+y=w659:dbl)
                }
                frame 20 {
                  n301 = call <vilib>:"Linear Fit.vi"("Y"=dbl[] [9.0, 10.0], "X"=dbl[] [9.187, 10.0]) -> ("slope"=w670:dbl, "intercept"=w668:dbl)  [unwired: 9 in, 3 out]
                  n302 = Multiply(x=w670, y=w669) -> (x*y=w667:dbl)
                  n303 = Add(x=w667, y=w668) -> (x+y=w666:dbl)
                }
                frame 21 {
                  n304 = call <vilib>:"Linear Fit.vi"("Y"=dbl[] [9.0, 10.0], "X"=dbl[] [9.187, 10.0]) -> ("slope"=w677:dbl, "intercept"=w675:dbl)  [unwired: 9 in, 3 out]
                  n305 = Multiply(x=w677, y=w676) -> (x*y=w674:dbl)
                  n306 = Add(x=w674, y=w675) -> (x+y=w673:dbl)
                }
                frame 22 {
                }
              }
            }
          }
          "Current" <- w486
          n307 = local read "Ring"() -> (w484:u16)
          n308 = case shown="1" w484 {
            tunnel: [w681 w686] -> w488
            tunnel: w487 -> [w681 w682]
            frame 0, Default {
            }
            frame 1 {
              # "channel 1일때 calibration"
              n309 = Threshold 1D Array(2:w682, 3:dbl[] [-11.0, -10.0, -9.0, -8.0, -7.0, -6.0, -5.0, -4.0, -3.0, -2.0, -1.0, 0.0, 1.0, 2.0, 3.0, 4.0, 5.0, 6.0, 7.0, 8.0, 9.0, 10.0, 11.0]) -> (0:w685:dbl)  [unwired: 1 in]
              n310 = Round Toward -Infinity(1:w685) -> (0:w683:dbl)
              n311 = case shown="2" w683 {
                tunnel: w682 -> [w687 w693 w700 w707 w714 w721 w728 w735 w742 w749 w754 w761 w768 w775 w782 w789 w796 w803 w810 w817 w824 w831 w835]
                tunnel: [w687 w690 w697 w704 w711 w718 w725 w732 w739 w746 w751 w758 w765 w772 w779 w786 w793 w800 w807 w814 w821 w828 w835] -> w686
                frame 0, Default {
                }
                frame 1 {
                  n312 = call <vilib>:"Linear Fit.vi"("Y"=dbl[] [-10.0, -9.0], "X"=dbl[] [-9.999, -9.19]) -> ("slope"=w694:dbl, "intercept"=w692:dbl)  [unwired: 9 in, 3 out]
                  n313 = Multiply(x=w694, y=w693) -> (x*y=w691:dbl)
                  n314 = Add(x=w691, y=w692) -> (x+y=w690:dbl)
                }
                frame 2 {
                  n315 = call <vilib>:"Linear Fit.vi"("Y"=dbl[] [-9.0, -8.0], "X"=dbl[] [-9.19, -8.169]) -> ("slope"=w701:dbl, "intercept"=w699:dbl)  [unwired: 9 in, 3 out]
                  n316 = Multiply(x=w701, y=w700) -> (x*y=w698:dbl)
                  n317 = Add(x=w698, y=w699) -> (x+y=w697:dbl)
                }
                frame 3 {
                  n318 = call <vilib>:"Linear Fit.vi"("Y"=dbl[] [-8.0, -7.0], "X"=dbl[] [-8.169, -7.149]) -> ("slope"=w708:dbl, "intercept"=w706:dbl)  [unwired: 9 in, 3 out]
                  n319 = Multiply(x=w708, y=w707) -> (x*y=w705:dbl)
                  n320 = Add(x=w705, y=w706) -> (x+y=w704:dbl)
                }
                frame 4 {
                  n321 = call <vilib>:"Linear Fit.vi"("Y"=dbl[] [-7.0, -6.0], "X"=dbl[] [-7.149, -6.128]) -> ("slope"=w715:dbl, "intercept"=w713:dbl)  [unwired: 9 in, 3 out]
                  n322 = Multiply(x=w715, y=w714) -> (x*y=w712:dbl)
                  n323 = Add(x=w712, y=w713) -> (x+y=w711:dbl)
                }
                frame 5 {
                  n324 = call <vilib>:"Linear Fit.vi"("Y"=dbl[] [-6.0, -5.0], "X"=dbl[] [-6.128, -5.106]) -> ("slope"=w722:dbl, "intercept"=w720:dbl)  [unwired: 9 in, 3 out]
                  n325 = Multiply(x=w722, y=w721) -> (x*y=w719:dbl)
                  n326 = Add(x=w719, y=w720) -> (x+y=w718:dbl)
                }
                frame 6 {
                  n327 = call <vilib>:"Linear Fit.vi"("Y"=dbl[] [-5.0, -4.0], "X"=dbl[] [-5.106, -4.084]) -> ("slope"=w729:dbl, "intercept"=w727:dbl)  [unwired: 9 in, 3 out]
                  n328 = Multiply(x=w729, y=w728) -> (x*y=w726:dbl)
                  n329 = Add(x=w726, y=w727) -> (x+y=w725:dbl)
                }
                frame 7 {
                  n330 = call <vilib>:"Linear Fit.vi"("Y"=dbl[] [-4.0, -3.0], "X"=dbl[] [-4.084, -3.062]) -> ("slope"=w736:dbl, "intercept"=w734:dbl)  [unwired: 9 in, 3 out]
                  n331 = Multiply(x=w736, y=w735) -> (x*y=w733:dbl)
                  n332 = Add(x=w733, y=w734) -> (x+y=w732:dbl)
                }
                frame 8 {
                  n333 = call <vilib>:"Linear Fit.vi"("Y"=dbl[] [-3.0, -2.0], "X"=dbl[] [-3.062, -2.04]) -> ("slope"=w743:dbl, "intercept"=w741:dbl)  [unwired: 9 in, 3 out]
                  n334 = Multiply(x=w743, y=w742) -> (x*y=w740:dbl)
                  n335 = Add(x=w740, y=w741) -> (x+y=w739:dbl)
                }
                frame 9 {
                  n336 = call <vilib>:"Linear Fit.vi"("Y"=dbl[] [-2.0, -1.0], "X"=dbl[] [-2.04, -1.018]) -> ("slope"=w750:dbl, "intercept"=w748:dbl)  [unwired: 9 in, 3 out]
                  n337 = Multiply(x=w750, y=w749) -> (x*y=w747:dbl)
                  n338 = Add(x=w747, y=w748) -> (x+y=w746:dbl)
                }
                frame 10 {
                  n339 = call <vilib>:"Linear Fit.vi"("Y"=dbl[] [-1.0, 0.0], "X"=dbl[] [-1.018, 0.004]) -> ("slope"=w755:dbl, "intercept"=w753:dbl)  [unwired: 9 in, 3 out]
                  n340 = Multiply(x=w755, y=w754) -> (x*y=w752:dbl)
                  n341 = Add(x=w752, y=w753) -> (x+y=w751:dbl)
                }
                frame 11 {
                  n342 = call <vilib>:"Linear Fit.vi"("Y"=dbl[] [0.0, 1.0], "X"=dbl[] [0.004, 1.025]) -> ("slope"=w762:dbl, "intercept"=w760:dbl)  [unwired: 9 in, 3 out]
                  n343 = Multiply(x=w762, y=w761) -> (x*y=w759:dbl)
                  n344 = Add(x=w759, y=w760) -> (x+y=w758:dbl)
                }
                frame 12 {
                  n345 = call <vilib>:"Linear Fit.vi"("Y"=dbl[] [1.0, 2.0], "X"=dbl[] [1.025, 2.047]) -> ("slope"=w769:dbl, "intercept"=w767:dbl)  [unwired: 9 in, 3 out]
                  n346 = Multiply(x=w769, y=w768) -> (x*y=w766:dbl)
                  n347 = Add(x=w766, y=w767) -> (x+y=w765:dbl)
                }
                frame 13 {
                  n348 = call <vilib>:"Linear Fit.vi"("Y"=dbl[] [2.0, 3.0], "X"=dbl[] [2.047, 3.069]) -> ("slope"=w776:dbl, "intercept"=w774:dbl)  [unwired: 9 in, 3 out]
                  n349 = Multiply(x=w776, y=w775) -> (x*y=w773:dbl)
                  n350 = Add(x=w773, y=w774) -> (x+y=w772:dbl)
                }
                frame 14 {
                  n351 = call <vilib>:"Linear Fit.vi"("Y"=dbl[] [3.0, 4.0], "X"=dbl[] [3.069, 4.09]) -> ("slope"=w783:dbl, "intercept"=w781:dbl)  [unwired: 9 in, 3 out]
                  n352 = Multiply(x=w783, y=w782) -> (x*y=w780:dbl)
                  n353 = Add(x=w780, y=w781) -> (x+y=w779:dbl)
                }
                frame 15 {
                  n354 = call <vilib>:"Linear Fit.vi"("Y"=dbl[] [4.0, 5.0], "X"=dbl[] [4.09, 5.112]) -> ("slope"=w790:dbl, "intercept"=w788:dbl)  [unwired: 9 in, 3 out]
                  n355 = Multiply(x=w790, y=w789) -> (x*y=w787:dbl)
                  n356 = Add(x=w787, y=w788) -> (x+y=w786:dbl)
                }
                frame 16 {
                  n357 = call <vilib>:"Linear Fit.vi"("Y"=dbl[] [5.0, 6.0], "X"=dbl[] [5.112, 6.133]) -> ("slope"=w797:dbl, "intercept"=w795:dbl)  [unwired: 9 in, 3 out]
                  n358 = Multiply(x=w797, y=w796) -> (x*y=w794:dbl)
                  n359 = Add(x=w794, y=w795) -> (x+y=w793:dbl)
                }
                frame 17 {
                  n360 = call <vilib>:"Linear Fit.vi"("Y"=dbl[] [6.0, 7.0], "X"=dbl[] [6.133, 7.154]) -> ("slope"=w804:dbl, "intercept"=w802:dbl)  [unwired: 9 in, 3 out]
                  n361 = Multiply(x=w804, y=w803) -> (x*y=w801:dbl)
                  n362 = Add(x=w801, y=w802) -> (x+y=w800:dbl)
                }
                frame 18 {
                  n363 = call <vilib>:"Linear Fit.vi"("Y"=dbl[] [7.0, 8.0], "X"=dbl[] [7.154, 8.174]) -> ("slope"=w811:dbl, "intercept"=w809:dbl)  [unwired: 9 in, 3 out]
                  n364 = Multiply(x=w811, y=w810) -> (x*y=w808:dbl)
                  n365 = Add(x=w808, y=w809) -> (x+y=w807:dbl)
                }
                frame 19 {
                  n366 = call <vilib>:"Linear Fit.vi"("Y"=dbl[] [8.0, 9.0], "X"=dbl[] [8.174, 9.195]) -> ("slope"=w818:dbl, "intercept"=w816:dbl)  [unwired: 9 in, 3 out]
                  n367 = Multiply(x=w818, y=w817) -> (x*y=w815:dbl)
                  n368 = Add(x=w815, y=w816) -> (x+y=w814:dbl)
                }
                frame 20 {
                  n369 = call <vilib>:"Linear Fit.vi"("Y"=dbl[] [9.0, 10.0], "X"=dbl[] [9.195, 10.0]) -> ("slope"=w825:dbl, "intercept"=w823:dbl)  [unwired: 9 in, 3 out]
                  n370 = Multiply(x=w825, y=w824) -> (x*y=w822:dbl)
                  n371 = Add(x=w822, y=w823) -> (x+y=w821:dbl)
                }
                frame 21 {
                  n372 = call <vilib>:"Linear Fit.vi"("Y"=dbl[] [9.0, 10.0], "X"=dbl[] [9.195, 10.0]) -> ("slope"=w832:dbl, "intercept"=w830:dbl)  [unwired: 9 in, 3 out]
                  n373 = Multiply(x=w832, y=w831) -> (x*y=w829:dbl)
                  n374 = Add(x=w829, y=w830) -> (x+y=w828:dbl)
                }
                frame 22 {
                }
              }
            }
          }
          "Voltage" <- w488
          n375 = Select(t="I mode" ("VI mode"), s=w494, f="V mode" ("VI mode")) -> (s? t:f=w502:string)
          n376 = property on="VI mode" class="Str"("Value"=w502) -> ()  [unwired: 2 in, 2 out]
          n377 = Pick Line(multi-line string="1A\n100mA\n10mA\n1mA\n100uA\n10uA\n1uA" ("Range"), line index=w495) -> (output string=w492:string)  [unwired: 1 in]
          n378 = case shown="\"1mA\"" w492 {
            tunnel: ["NONE" w840 w848 w856 w864 w872 w880 w888] -> w491
            tunnel: w486 -> [_ w839 w845 w855 w863 w871 w879 w887]
            frame "False", Default {
            }
            frame "100mA" {
              n379 = Multiply(x=w839, y=100.0) -> (x*y=w843:dbl)
              n380 = Divide(x=w843, y=10.0) -> (x/y=w838:dbl)
              n381 = Number To Fractional String(number=w838) -> (F-format string=w837:string)  [unwired: 3 in]
              n382 = Concatenate Strings(w837, "mA" ("string")) -> (w840:string)
            }
            frame "10mA" {
              n383 = Multiply(x=w845, y=10.0) -> (x*y=w851:dbl)
              n384 = Divide(x=w851, y=10.0) -> (x/y=w847:dbl)
              n385 = Number To Fractional String(number=w847) -> (F-format string=w846:string)  [unwired: 3 in]
              n386 = Concatenate Strings(w846, "mA" ("string")) -> (w848:string)
            }
            frame "1mA" {
              n387 = Multiply(x=w855, y=1.0) -> (x*y=w859:dbl)
              n388 = Divide(x=w859, y=10.0) -> (x/y=w854:dbl)
              n389 = Number To Fractional String(number=w854) -> (F-format string=w853:string)  [unwired: 3 in]
              n390 = Concatenate Strings(w853, "mA" ("string")) -> (w856:string)
            }
            frame "100uA" {
              n391 = Multiply(x=w863, y=100.0) -> (x*y=w867:dbl)
              n392 = Divide(x=w867, y=10.0) -> (x/y=w862:dbl)
              n393 = Number To Fractional String(number=w862) -> (F-format string=w861:string)  [unwired: 3 in]
              n394 = Concatenate Strings(w861, "uA" ("string")) -> (w864:string)
            }
            frame "10uA" {
              n395 = Multiply(x=w871, y=10.0) -> (x*y=w875:dbl)
              n396 = Divide(x=w875, y=10.0) -> (x/y=w870:dbl)
              n397 = Number To Fractional String(number=w870) -> (F-format string=w869:string)  [unwired: 3 in]
              n398 = Concatenate Strings(w869, "uA" ("string")) -> (w872:string)
            }
            frame "1uA" {
              n399 = Multiply(x=w879, y=1.0) -> (x*y=w884:dbl)
              n400 = Divide(x=w884, y=10.0) -> (x/y=w878:dbl)
              n401 = Number To Fractional String(number=w878) -> (F-format string=w877:string)  [unwired: 3 in]
              n402 = Concatenate Strings(w877, "uA" ("string")) -> (w880:string)
            }
            frame "1A" {
              n403 = Multiply(x=w887, y=1.0) -> (x*y=w891:dbl)
              n404 = Divide(x=w891, y=10.0) -> (x/y=w886:dbl)
              n405 = Number To Fractional String(number=w886) -> (F-format string=w885:string)  [unwired: 3 in]
              n406 = Concatenate Strings(w885, "A" ("string")) -> (w888:string)
            }
          }
          n407 = property on="Range" class="Str"("Value"=w492) -> ()  [unwired: 2 in, 2 out]
          n408 = Bundle("trimmed string"=w501, "Enable"=w503, "VI mode"=w502, "output string"=w492, w489, w488, w486, w491) -> (w525:T2)  [unwired: 1 in]
        }
        "Array 2" <- w426
        "Array 3" <- w425
        "Array" <- w405
        n409 = local read "Ring"() -> (w427:u16)
        n410 = Decrement(x=w427) -> (x-1=w411:u16)
        n411 = Index Array(array=w426, index=w411) -> (element=w413:i32)
        n412 = Index Array(array=w425, index=w411) -> (element=w414:bool)
        n413 = Index Array(array=w416, index=w411) -> (element=w415:bool)
        n414 = Index Array(array=w412, index=w411) -> (element=w410:dbl)
        n415 = case shown="True" w409 {
          selector: w409 -> [w429 _]
          tunnel: w415 -> [_ w434]
          tunnel: w414 -> [_ w433]
          tunnel: w413 -> [_ w432]
          tunnel: w410 -> [_ w431]
          tunnel: [w429 FALSE] -> w408
          frame False {
          }
          frame True {
            n416 = local write "Enable"(w434) -> ()
            n417 = local write "Mode"(w433) -> ()
            n418 = local write "Range"(w432) -> ()
            n419 = local write "Output Value"(w431) -> ()
          }
        }
        n420 = case shown="3" w413 {
          tunnel: ["mA" "mA" "mA" "uA" "uA" "uA" "nA"] -> w423
          frame 0, Default {
          }
          frame 1 {
          }
          frame 2 {
          }
          frame 3 {
          }
          frame 4 {
          }
          frame 5 {
          }
          frame 6 {
          }
        }
        n421 = Select(t=w423, s=w414, f="V") -> (s? t:f=w424:string)
        n422 = local write "Unit"(w424) -> ()
      }
      frame True {
        n423 = property on="String" class="Str"() -> ("Value"=w897:string)  [unwired: 2 in, 2 out]
        n424 = VISA Write(VISA resource name=w898, write buffer=w897) -> (VISA resource name out=w895:refnum<visa-resource-name>, error out=w896:errorcluster)  [unwired: 1 in, 1 out]
        n425 = property on="Write mode" class="Bool (strict)"(error in=w896, "Value"=FALSE ("Write mode")) -> (error out=w894:errorcluster)  [unwired: 1 in, 1 out]
      }
    }
  }
  n426 = VISA Close(VISA resource name=w18, error in (no error)=w12) -> (error out=w11:errorcluster)
  n427 = call <vilib>:"Simple Error Handler.vi"("error in (no error)"=w11) -> ()  [unwired: 4 in, 5 out]
